vi "WriteToDAC.vi"(4 "converter box version":i16=2, 5 "DAC New Reset":bool, 6 "New DAC values generated":T1 {"bit index" min=-1 max=17 step=1; "channel index" max=7 step=1; "offset" max=4095; "DAC voltage"."ch1" max=4095 step=1; "DAC voltage"."ch0" max=4095 step=1}, 7 "DAC values to write In":T1 {"bit index" min=-1 max=17 step=1; "channel index" max=7 step=1; "offset" max=4095; "DAC voltage"."ch1" max=4095 step=1; "DAC voltage"."ch0" max=4095 step=1}, 8 "DAC Reset State In":bool) -> (2 "DAC values to write out":T1 {"bit index" min=-1 max=17 step=1; "channel index" max=7 step=1; "offset" max=4095; "DAC voltage"."ch1" max=4095 step=1; "DAC voltage"."ch0" max=4095 step=1}, 3 "DAC Reset State out":bool)   [LabVIEW 2010]
uses:
  FPGA_Typedefs/DAC_values_cluster.ctl
  FPGA_Typedefs/DAC_voltage_cluster.ctl
  <vilib>/eio/EIONode/EIONode.xnode
  <vilib>/rvi/eio/nirviEIOImplementation/nirviEIOImplementation.xnode
  <vilib>/rvi/eio/common/nirviEmuClasses.ctl
  <vilib>/rvi/eio/common/nirviEmuTemplateMethod_noerrors.vi
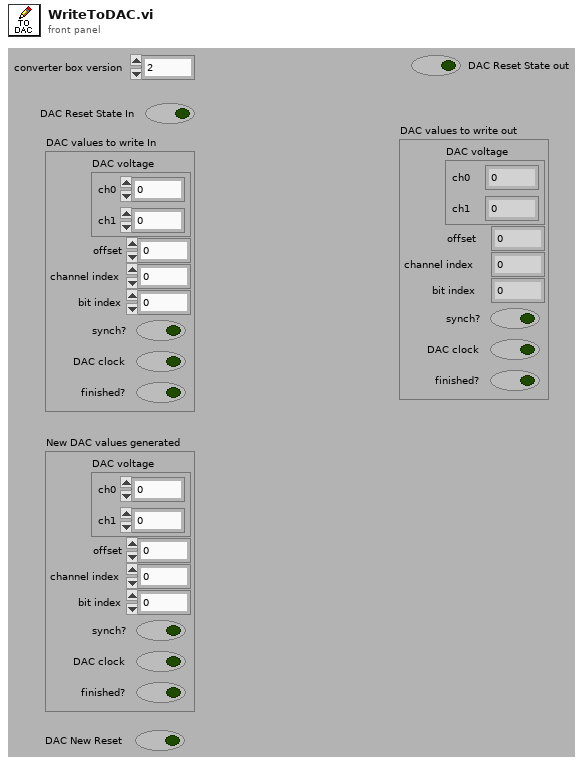
[diagram p1: front panel]
types:
  T1 = typedef "DAC_values_cluster.ctl" = cluster{"DAC voltage":T2, "offset":u16, "channel index":u16, "bit index":i32, "synch?":bool, "DAC clock":bool, "finished?":bool}
  T2 = typedef "DAC_voltage_cluster.ctl" = cluster{"ch0":u16, "ch1":u16}
  T3 = typedef "nirviEmuClasses.ctl" = enum16{"IO Read", "IO Write", "Method", "Property Read", "Property Write"}
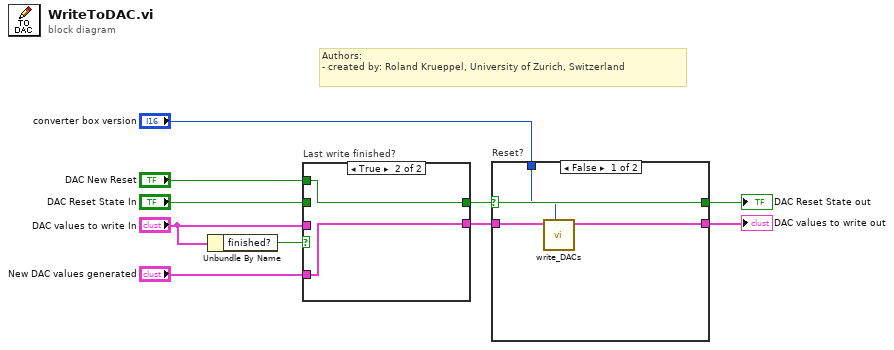
[diagram p0: block diagram]
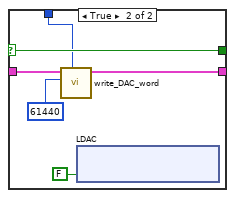
[diagram p2: hidden frame]
diagram:
  # "Authors: \n- created by: Roland Krueppel, University of Zurich, Switzerland"
  n1 = Unbundle By Name("DAC values to write In") -> ("finished?"=w7:bool)
  n2 = case "Last write finished?" shown="True" w7 {
    tunnel: "DAC Reset State In" -> [w11 _]
    tunnel: "DAC values to write In" -> [w12 _]
    tunnel: "New DAC values generated" -> [_ w14]
    tunnel: [w12 w14] -> w3
    tunnel: [w11 w13] -> w2
    tunnel: "DAC New Reset" -> [_ w13]
    frame False {
    }
    frame True {
    }
  }
  n3 = case "Reset?" shown="False" w2 {
    selector: w2 -> [w17 w21]
    tunnel: [w18 w22] -> w5
    tunnel: [w17 w21] -> w6
    tunnel: "converter box version" -> [w16 w20]
    tunnel: w3 -> [w15 w19]
    frame False {
      n4 = call "write_DACs.vi"("converter box version"=w16, "DAC values in"=w15) -> ("DAQ values out"=w18:T1)  [unwired: 9 in]
    }
    frame True {
      n5 = call "write_DAC_word.vi"("converter box version"=w20, "U16 data number"=u16 61440, "DAC values in"=w19) -> ("DAC values out"=w22:T1)  [unwired: 8 in]
      n6 = xnode "LDAC"("Connector1/DIO32"=FALSE ("LDAC")) -> ()  [unwired: 1 in, 1 out]
    }
  }
  "DAC Reset State out" <- w6
  "DAC values to write out" <- w5
